vi "Bool 1D.vi"(4 "Array":bool[](array[boolean])) -> (1 "Abs_Boolean_1D.lvclass":refnum<class "Abs_Boolean_1D.lvclass">)   [LabVIEW 2021, in "Const_Bool_1D.lvclass"]
uses:
  Const_Bool_1D.lvclass
  Abs_Types/Boolean_1D/Abs_Boolean_1D.lvclass
  C:/TSA/LV_Abstract/Source/Abs_Types/Boolean_1D/Abs_Boolean_1D.lvclass
  Const_Bool_1D.lvclass/Const_Bool_1D.ctl
  Properties/Write Value.vi
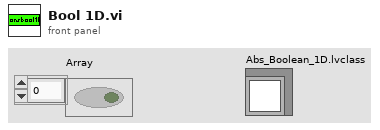
[diagram p1: front panel]
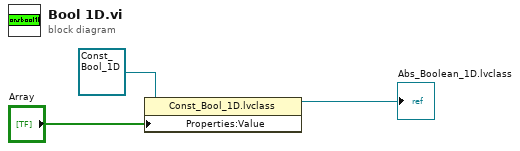
[diagram p0: block diagram]
diagram:
  n1 = property class="Const_Bool_1D.lvclass"(reference=refnum<class "Const_Bool_1D.lvclass"> refnum ("Constants.lvlib:Boolean.lvclass"), "Properties:Value"="Array") -> (reference out=→"Abs_Boolean_1D.lvclass":refnum<class "Const_Bool_1D.lvclass">)  [unwired: 1 in, 1 out]
